vi "updata LeafNumber for traverse.vi"(8 "error in":errorcluster caption="错误输入（无错误）", 10 "Data in":u8, 11 "Class in":refnum<class "PanelLinkNode.lvclass"> caption="DNL_LabVIEW Object in") -> (0 "error out":errorcluster caption="错误输出", 1 "Stop Traverse":bool, 2 "Data out":u8, 3 "Class out":refnum<class "PanelLinkNode.lvclass"> caption="DNL_LabVIEW Object out")   [LabVIEW 2016, in "PanelLinkNode.lvclass"]
uses:
  PanelLinkNode.lvclass
  PanelLinkNode.lvclass/PanelLinkNode.ctl
panel:
  # "将该控件替换成所需的数据类型控件"
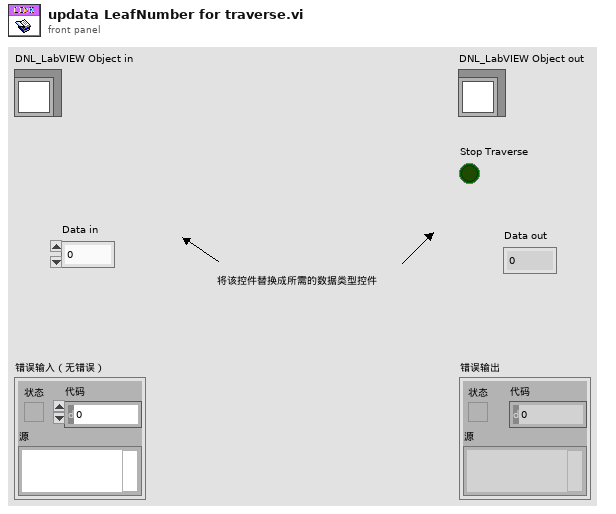
[diagram p1: front panel]
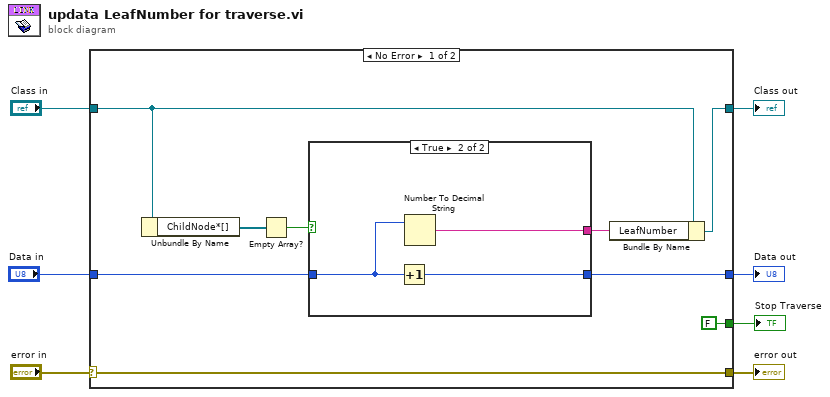
[diagram p0: block diagram]
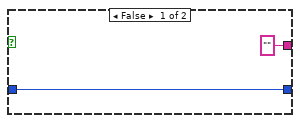
[diagram p2: hidden frame]
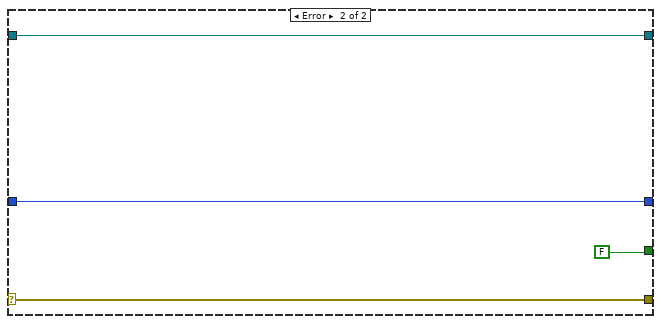
[diagram p3: hidden frame]
diagram:
  n1 = case shown="No Error" "error in" {
    selector: "error in" -> [w16 w25]
    tunnel: [w16 w25] -> w6
    tunnel: [w9 w24] -> w4
    tunnel: "Class in" -> [w10 w24]
    tunnel: "Data in" -> [w12 w23]
    tunnel: [w11 w23] -> w2
    tunnel: [FALSE FALSE] -> w1
    frame No Error {
      n2 = Unbundle By Name(w10) -> ("ChildNode*[]"=w14:refnum<data-value>[])
      n3 = Empty Array?(array=w14) -> (empty?=w13:bool)
      n4 = case shown="True" w13 {
        tunnel: w12 -> [w17 w20]
        tunnel: [w17 w21] -> w11
        tunnel: ["" w19] -> w8
        frame False {
        }
        frame True {
          n5 = Increment(x=w20) -> (x+1=w21:u8)
          n6 = Number To Decimal String(number=w20) -> (decimal integer string=w19:string)  [unwired: 1 in]
        }
      }
      n7 = Bundle By Name(cluster=w10, "LeafNumber"=w8) -> (w9:refnum<class "PanelLinkNode.lvclass">)
    }
    frame Error {
    }
  }
  "error out" <- w6
  "Class out" <- w4
  "Data out" <- w2
  "Stop Traverse" <- w1
